vi "Construct.vi"(0 "Export Config File":path, 1 "Component Root Path":path) -> (4 "Export Out":refnum<class "Export.lvclass">)   [LabVIEW 2017, in "CL_G3_VIComponentBuilder.lvlib" / "Export.lvclass"]
doc: "Brings the Export object into existence and sets the initial values according to the Export Config File."
uses:
  Export.lvclass
  Export.lvclass/Export.ctl
  Accessors/Write Export Config File.vi
  Accessors/Write Component Root path.vi
  Accessors/Write Export Operation Errors.vi
  <vilib>/Utility/libraryn.llb/Check if File or Folder Exists.vi
  <vilib>/Utility/error.llb/Error Cluster From Error Code.vi
  <vilib>/Utility/config.llb/NI_LVConfig.lvlib
  CL_G3_VIComponentBuilder.lvlib
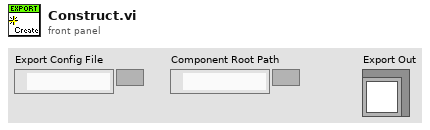
[diagram p1: front panel]
types:
  T1 = typedef "NI_LVConfig.lvlib/Config Data RefNum.ctl" = refnum<k1>
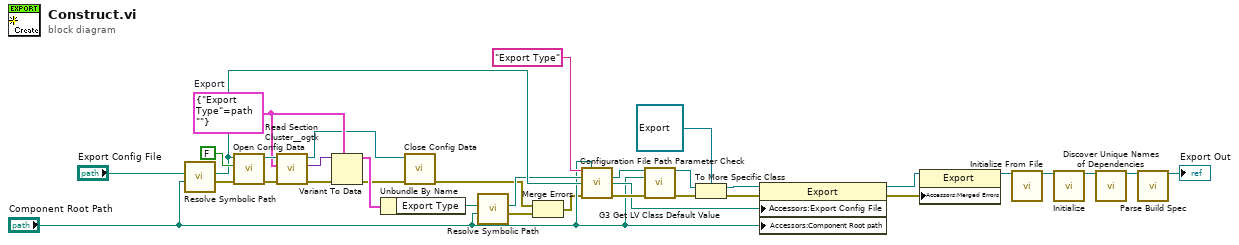
[diagram p0: block diagram]
diagram:
  w24 = cluster{"Export Type":path} {"Export Type"=path ""}  # Export
  n1 = call "Resolve Symbolic Path.vi"("Component Root Path"="Component Root Path", "Path In"="Export Config File") -> ("error out"=w7:errorcluster, "Path Out"=w15:path)  [unwired: 8 in]
  n2 = call <vilib>:"Open Config Data.vi"("error in (no error)"=w7, "create file if necessary (T)"=FALSE, "configuration file path"=w15) -> ("error out"=w22:errorcluster, "refnum"=w27:T1)  [unwired: 6 in, 1 out]
  n3 = call <userlib>:"Read Section Cluster__ogtk.vi"("error in (no error)"=w22, "Section Formatted Cluster Type"=w24, "refnum"=w27) -> ("error out"=w21:errorcluster, "Section Formatted Cluster"=w26:variant, "dup refnum"=w23:T1)  [unwired: 4 in, 2 out]
  n4 = Variant To Data(error in=w21, type=w24, Variant=w26) -> (data=w25:cluster{"Export Type":path}, error out=w20:errorcluster)
  n5 = Unbundle By Name(w25) -> ("Export Type"=w6:path)
  n6 = call <vilib>:"Close Config Data.vi"("error in (no error)"=w20, "refnum"=w23) -> ("error out"=w3:errorcluster)  [unwired: 8 in, 1 out]
  n7 = call "Resolve Symbolic Path.vi"("Component Root Path"="Component Root Path", "Path In"=w6) -> ("error out"=w2:errorcluster, "Path Out"=w5:path)  [unwired: 8 in]
  n8 = Merge Errors(w3, w2) -> (w1:errorcluster)
  n9 = call "Configuration File Path Parameter Check.vi"("Parameter Name"="Export Type", "Component Root Path"="Component Root Path", "Specified Path in Configuration File"=w5, "Configuration File Path"=w15, "error in (no error)"=w1) -> ("dup Specified Path in Configuration File"=w12:path, "dup Configuration File Path"=w13:path, "error out"=w14:errorcluster)  [unwired: 8 in]
  n10 = call "G3 Get LV Class Default Value.vi"("Export Type"=w12, "Component Definition ini Path"="Component Root Path", "error in (no error)"=w14) -> ("LabVIEW Object out"=w34:refnum<class>, "error out"=w33:errorcluster)  [unwired: 11 in]
  n11 = To More Specific Class(target class=refnum<class "Export.lvclass"> refnum ("Export Out"), reference=w34, error in=w33) -> (specific class reference=w31:refnum<class "Export.lvclass">, error out=w8:errorcluster)
  n12 = property class="Export"(reference=w31, error in=w8, "Accessors:Export Config File"=w13, "Accessors:Component Root path"="Component Root Path") -> (reference out=w29:refnum<class "Export.lvclass">, error out=w9:errorcluster)
  n13 = property class="Export"(reference=w29, "Accessors:Merged Errors"=w9) -> (reference out=w10:refnum<class "Export.lvclass">)  [unwired: 1 in, 1 out]
  n14 = call-dynamic "Initialize From File.vi"("Export in"=w10) -> ("Export out"=w11:refnum<class "Export.lvclass">)  [unwired: 14 in]
  n15 = call-dynamic "Initialize.vi"("Export in"=w11) -> ("Export out"=w30:refnum<class "Export.lvclass">)  [unwired: 14 in]
  n16 = call-dynamic "Discover Unique Names of Dependencies.vi"("Export In"=w30) -> ("Export Out"=w19:refnum<class "Export.lvclass">)  [unwired: 14 in]
  n17 = call-dynamic "Parse Build Spec.vi"("Export In"=w19) -> ("Export Out"=→"Export Out":refnum<class "Export.lvclass">)  [unwired: 14 in]
